vi "loadDataNodeBegin.vi"(8 "error in (no error)":errorcluster, 10 "XML Refnum in":refnum<file>, 11 "Void in":refnum<class "Void.lvclass">) -> (0 "error out":errorcluster, 2 "XML Refnum out":refnum<file>, 3 "Void out":refnum<class "Void.lvclass">)   [LabVIEW 2013, in "Void.lvclass"]
doc: "Part of the file loading process. Occurs at the beginning of a node being loaded. Loads the common xceDataNode data name and description."
uses:
  Void.lvclass
  xCE/xceNode/xceNode.lvclass
  XML Parser/XML Parser.lvclass
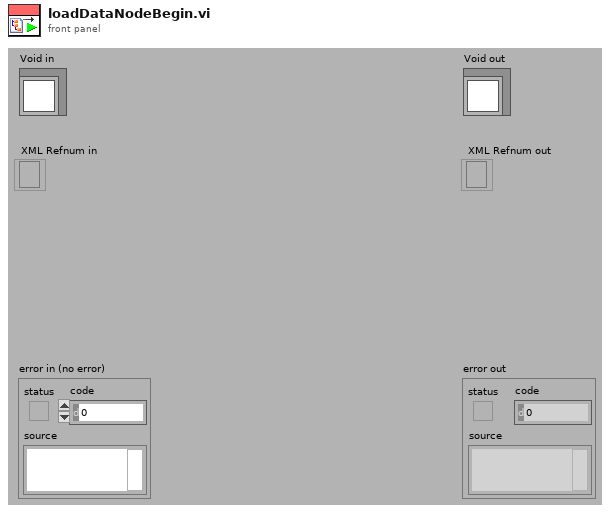
[diagram p1: front panel]
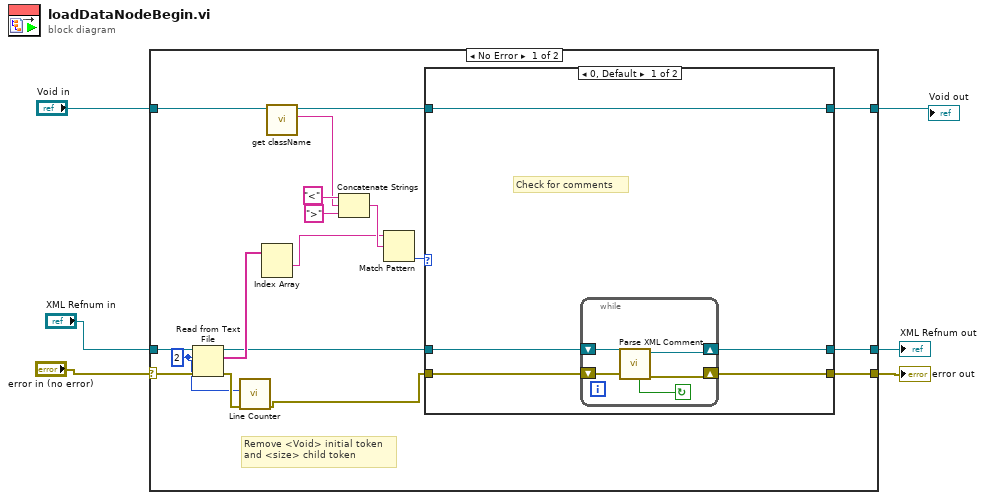
[diagram p0: block diagram]
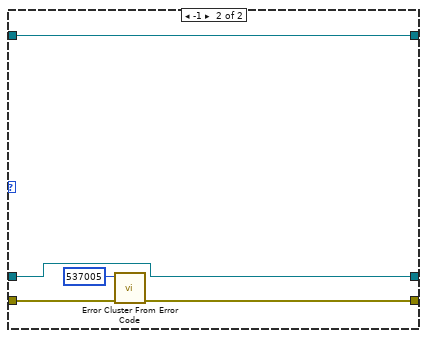
[diagram p2: hidden frame]
diagram:
  n1 = case shown="No Error" "error in (no error)" {
    selector: "error in (no error)" -> [w24 w42]
    tunnel: [w14 w42] -> w2
    tunnel: [w10 w41] -> w1
    tunnel: "Void in" -> [w21 w41]
    tunnel: "XML Refnum in" -> [w23 w40]
    tunnel: [w11 w40] -> w3
    frame No Error {
      w8 = 2 ("count")
      # "Remove <Void> initial token\nand <size> child token"
      n2 = Read from Text File(file (use dialog)=w23, count=w8, error in=w24) -> (refnum out=w12:refnum<file>, text=w22:string[], error out=w9:errorcluster)  [unwired: 1 in, 1 out]
      n3 = call "Line Counter.vi"("error in (no error)"=w9, "# of lines to increment (1)"=w8) -> ("error out"=w7:errorcluster)  [unwired: 8 in, 1 out]
      n4 = Index Array(array=w22) -> (element #1=w16:string)  [unwired: 2 in, 1 out]
      n5 = call "get className.vi"("xceNode in"=w21) -> ("Class name"=w19:string, "xceNode out"=w13:refnum<class "Void.lvclass">)  [unwired: 8 in, 1 out]
      n6 = Concatenate Strings("<", w19, ">" ("string")) -> (w17:string)
      n7 = Match Pattern(string=w16, regular expression=w17) -> (offset past match=w15:i32)  [unwired: 1 in, 3 out]
      n8 = case shown="0, Default" w15 {
        tunnel: w7 -> [w27 w39]
        tunnel: [w26 w38] -> w14
        tunnel: w13 -> [w29 w35]
        tunnel: w12 -> [w28 w36]
        tunnel: [w25 w36] -> w11
        tunnel: [w29 w35] -> w10
        frame 0, Default {
          # "Check for comments"
          n9 = while {
            shift-right: [w30] -> w25
            shift-left: w28 -> [w34]
            shift-right: [w31] -> w26
            shift-left: w27 -> [w33]
            stop <- w32 continue-if-true
            n10 = call "Parse XML Comment.vi"("error in (no error)"=w33, "XML Refnum in"=w34) -> ("error out"=w31:errorcluster, "XML Refnum out"=w30:refnum<file>, "Comment Line Found"=w32:bool)  [unwired: 6 in, 1 out]
          }
        }
        frame -1 {
          n11 = call <vilib>:"Error Cluster From Error Code.vi"("error in (no error)"=w39, "error code (0)"=537005) -> ("error out"=w38:errorcluster)  [unwired: 7 in]
        }
      }
    }
    frame Error {
    }
  }
  "error out" <- w2
  "Void out" <- w1
  "XML Refnum out" <- w3
